vi "Library - Properties.vi"(7 "Msg Chain":string, 8 "error in (no error)":errorcluster {"code" format="Error %.0f"}, 10 "Libraries":refnum<class "Library Documentation.lvclass">[](array[class]), 11 "VIDoc Printer - Confluence In":refnum<class "VIDoc Printer - Confluence.lvclass">) -> (0 "error out":errorcluster {"code" format="Error %.0f"}, 3 "VIDoc Printer - Confluence Out":refnum<class "VIDoc Printer - Confluence.lvclass">)   [LabVIEW 2023, in "VIDoc Printer - Confluence.lvlib" / "VIDoc Printer - Confluence.lvclass"]
uses:
  VIDoc Printer - Confluence.lvclass
  C:/projects/DMC/Tooling/Git-Action-Service/Source/Documentation Generation/Printers/Printer/VIDoc Printer.lvclass
  Parsing/Library Documentation/Library Documentation.lvclass
  Parsing/Library Documentation/Library Documentation.lvclass/Library Documentation.ctl
  Confluence Formatting/Types/Format Combo Box.ctl
  VIDoc Printer - Confluence.lvclass/VIDoc Printer - Confluence.ctl
  Parsing/Library Documentation/Get Path.vi
  Parsing/Library Documentation/Get Library Info.vi
  Parsing/Library Documentation/Get Name.vi
  Parsing/Library Documentation/Get Total Data Size.vi
  Printer/VIDoc Printer.lvclass
  UI Interaction/UI Interaction.lvclass
  Confluence Formatting/Confluence Formatting.lvlib
  C:/projects/DMC/Tooling/Git-Action-Service/Source/Documentation Generation/Printers/Confluence Printer/VIDoc Printer - Confluence.lvclass
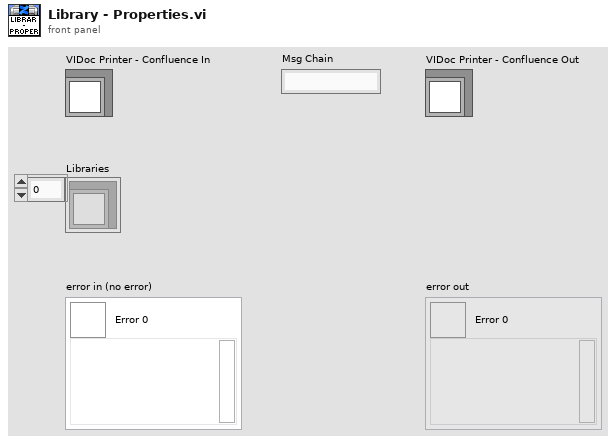
[diagram p1: front panel]
types:
  T1 = typedef "Confluence Formatting.lvlib/Format Combo Box.ctl" = string
  T2 = typedef "VIDoc Parsing.lvlib/Base Library Info Cluster.ctl" = cluster{"Name":string, "Icon":T3, "Version":cluster{"Major":u16, "Minor":u16, "Fix":u16, "Build":u16}, "Description":string, "Path":path, "Friends":string[], "Library Scope":enum32{"invalid scope", "public", "private", "protected", "community"}, "Qualified Name":string}
  T3 = typedef "imagedata.ctl" = cluster{"image type":i32, "image depth":i32, "image":u8[], "mask":u8[], "colors":u32[], "Rectangle":cluster{"left":i16, "top":i16, "right":i16, "bottom":i16}}
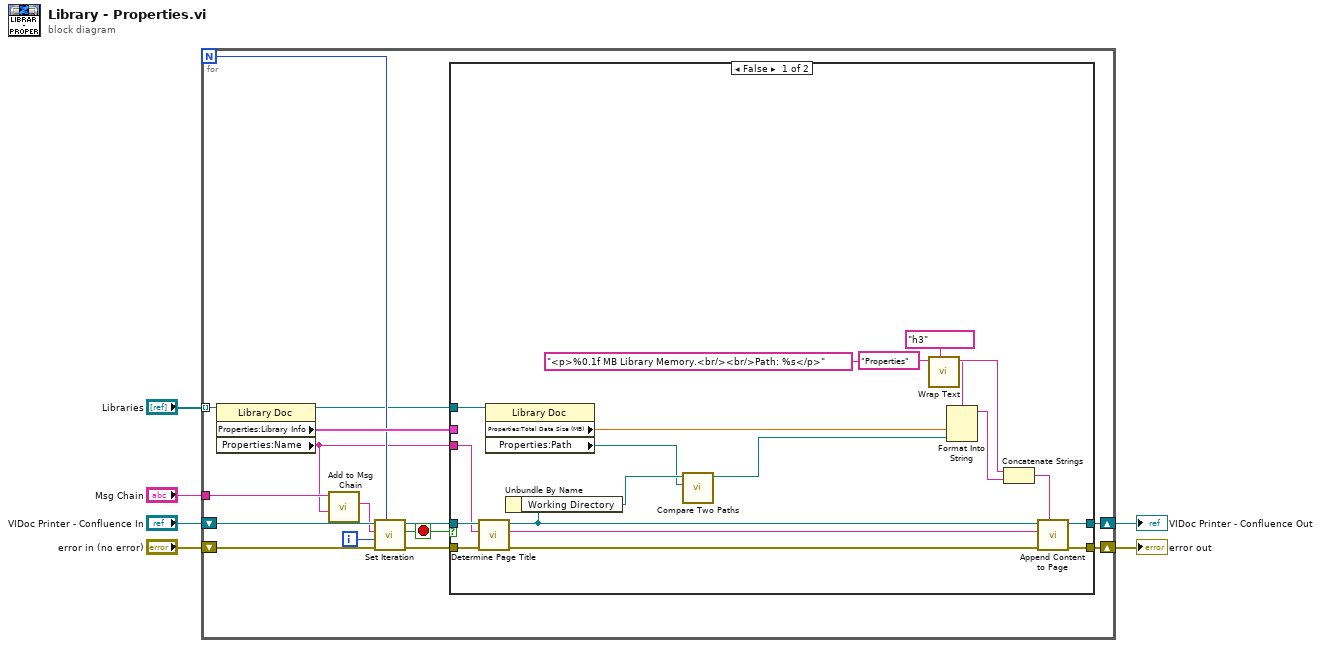
[diagram p0: block diagram]
diagram:
  n1 = for {
    N -> [w13]
    shift-right: [w19] -> w6
    shift-left: "error in (no error)" -> [w16]
    shift-right: [w20] -> w5
    shift-left: "VIDoc Printer - Confluence In" -> [w17]
    tunnel: "Libraries" -> [w21] mode=indexing
    tunnel: "Msg Chain" -> [w11]
    i -> [w12]
    stop <- w8 stop-if-true
    n2 = property class="Library Doc"(reference=w21) -> (reference out=w7:refnum<class "Library Documentation.lvclass">, "Properties:Library Info"=w18:T2, "Properties:Name"=w10:string)  [unwired: 1 in, 1 out]
    n3 = call "Add to Msg Chain.vi"("New"=w10, "Msg Chain in"=w11) -> ("Msg Chain out"=w9:string)  [unwired: 9 in]
    n4 = call "Set Iteration.vi"("Progress Max"=w13, "error in (no error)"=w16, "Progress Value"=w12, "Message (No Message Update)"=w9, "VIDoc Printer In"=w17) -> ("error out"=w14:errorcluster, "Abort?"=w8:bool, "VIDoc Printer Out"=w15:refnum<class "VIDoc Printer - Confluence.lvclass">)  [unwired: 4 in]
    n5 = case shown="False" w8 {
      tunnel: [w38 w41] -> w20
      tunnel: [w37 w42] -> w19
      tunnel: w18 -> [_ _]
      tunnel: w15 -> [w33 w41]
      tunnel: w14 -> [w32 w42]
      tunnel: w10 -> [w31 _]
      tunnel: w7 -> [w27 _]
      frame False {
        n6 = call "Determine Page Title.vi"("error in (no error)"=w32, "Name"=w31, "VIDoc Printer - Confluence In"=w33) -> ("error out"=w39:errorcluster, "Page Title"=w40:string, "VIDoc Printer - Confluence Out"=w25:refnum<class "VIDoc Printer - Confluence.lvclass">)  [unwired: 5 in, 1 out]
        n7 = property class="Library Doc"(reference=w27) -> ("Properties:Total Data Size (MB)"=w29:dbl, "Properties:Path"=w23:path)  [unwired: 1 in, 2 out]
        n8 = Unbundle By Name(w25) -> ("Working Directory"=w24:path)
        n9 = call <vilib>:"Compare Two Paths.vi"("Path 2"=w23, "Path 1"=w24) -> ("Relative Path from 1 to 2"=w22:path)  [unwired: 6 in, 3 out]
        n10 = call "Wrap Text.vi"("Formatting"=T1 "h3", "String"="Properties") -> ("Wrapped String"=w35:string)  [unwired: 8 in, 1 out]
        n11 = Format Into String(format string="<p>%0.1f MB Library Memory.<br/><br/>Path: %s</p>", w29, w22) -> (resulting string=w26:string)  [unwired: 2 in, 1 out]
        n12 = Concatenate Strings(w35, w26) -> (w34:string)
        n13 = call "Append Content to Page.vi"("Page Content"=w34, "error in (no error)"=w39, "Page Title"=w40, "VIDoc Printer - Confluence In"=w25) -> ("error out"=w37:errorcluster, "VIDoc Printer - Confluence Out"=w38:refnum<class "VIDoc Printer - Confluence.lvclass">)  [unwired: 6 in]
      }
      frame True {
      }
    }
  }
  "error out" <- w6
  "VIDoc Printer - Confluence Out" <- w5
